vi "Get_Ch_data_from_file.vi"(0 "Filename":path, 9 "Channel names":string[](array[string]), 11 "Start of read offset (chars.: 0)":i32, 12 "Averaging Time(s)":dbl=5.0) -> (4 "exists?":bool, 6 "File Channels":string[](array[string]), 10 "Times":dbl[](array[numeric]) format="%.2f", 15 "Ch Data":dbl[][](array[numeric]) format="%.2f")   [LabVIEW 2015]
uses:
  <vilib>/Analysis/baseanly.llb/Mean (DBL).vi
  <vilib>/Analysis/NI_AALBase.lvlib
panel:
  in  "stop":bool
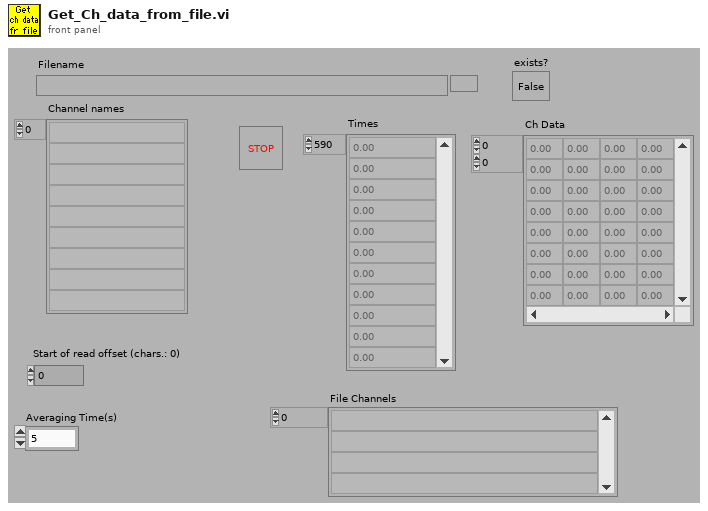
[diagram p1: front panel]
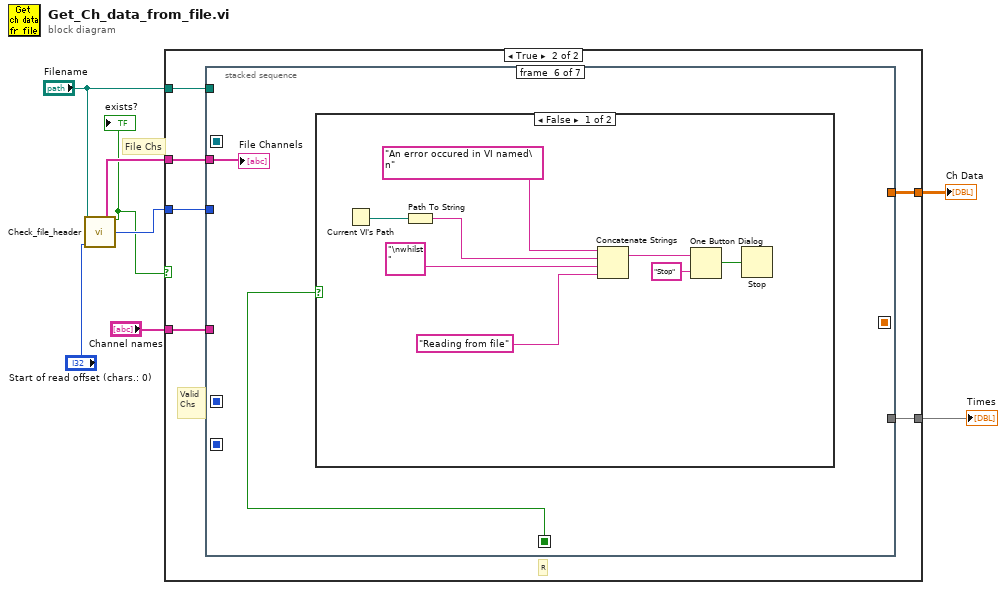
[diagram p0: block diagram]
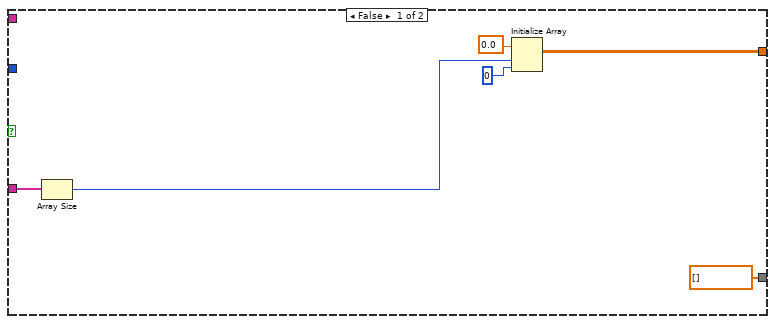
[diagram p2: hidden frame]
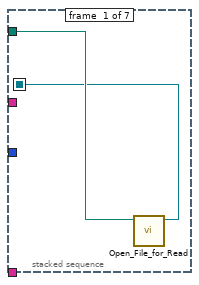
[diagram p3: hidden frame]
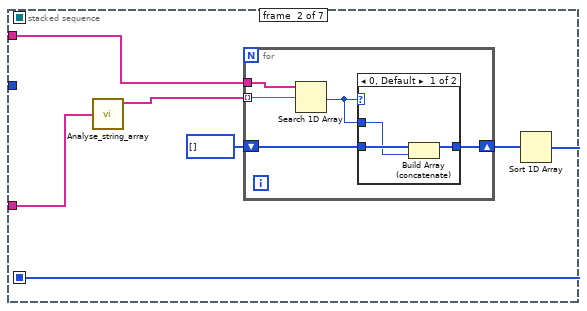
[diagram p4: hidden frame]
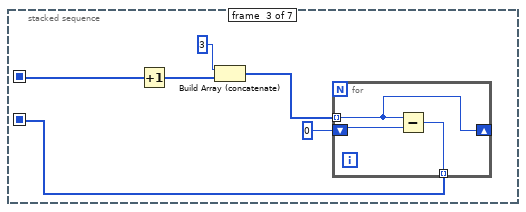
[diagram p6: hidden frame]
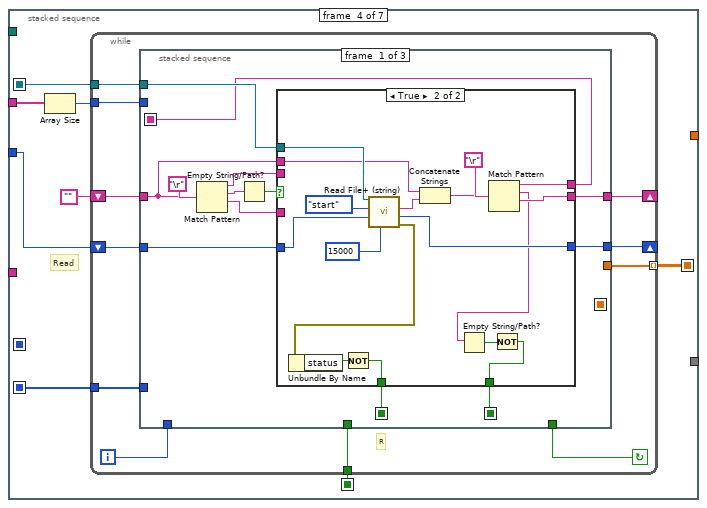
[diagram p7: hidden frame]
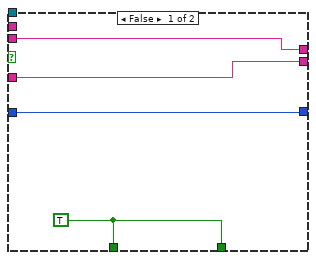
[diagram p8: hidden frame]
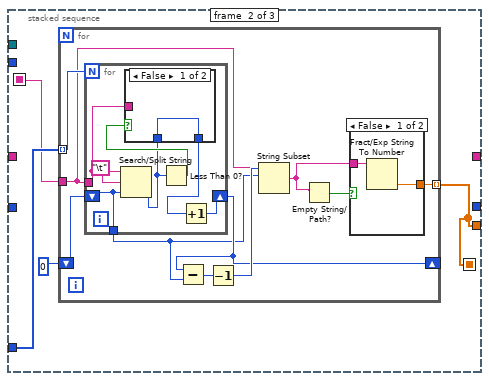
[diagram p9: hidden frame]
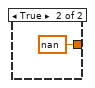
[diagram p10: hidden frame]
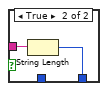
[diagram p11: hidden frame]
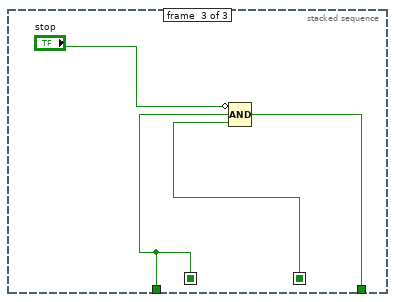
[diagram p12: hidden frame]
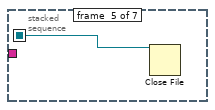
[diagram p13: hidden frame]
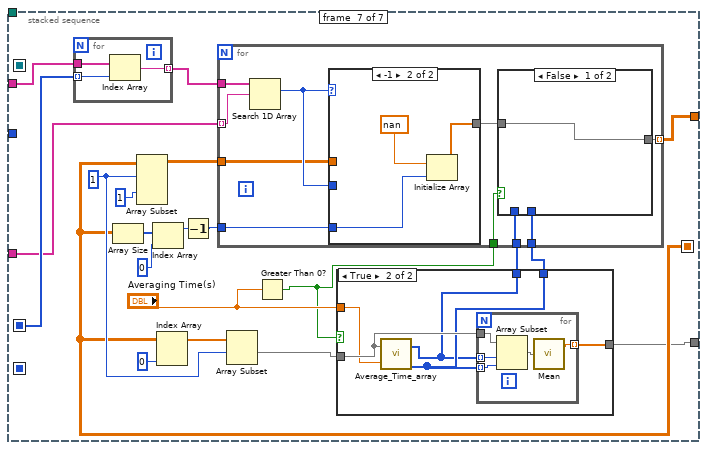
[diagram p15: hidden frame]
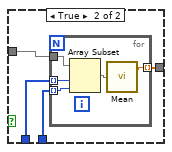
[diagram p17: hidden frame]
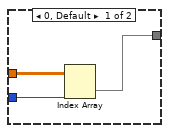
[diagram p18: hidden frame]
diagram:
  # "File Chs"
  n1 = call "Check_file_header.vi"("Filename"="Filename", "Start of read offset (chars.: 0)"="Start of read offset (chars.: 0)") -> ("File Channels"=w7:string[], "exists?"=w4:bool, "Start of data (bytes)"=w8:i32)  [unwired: 2 in, 9 out]
  "exists?" <- w4
  n2 = case shown="True" w4 {
    tunnel: w8 -> [_ w19]
    tunnel: w7 -> [_ w18]
    tunnel: "Filename" -> [_ w20]
    tunnel: [w9 w16] -> w3
    tunnel: [dbl[] [] w15] -> w2
    tunnel: "Channel names" -> [w11 w17]
    frame False {
      n3 = Array Size(array=w11) -> (size(s)=w10:i32)
      n4 = Initialize Array(0.0, w10, 0 ("Dimension Size")) -> (w9:dbl[][])
    }
    frame True {
      # "Valid\nChs"
      # "R"
      n5 = stacked-sequence {
        seq-local: [w21 _ _ _ _ _ _] -> [_ _ _ w53 w131 _ _]
        seq-local: [_ _ _ w50 _ _ _] -> [_ _ _ _ _ w133 _]
        seq-local: [_ _ _ w48 _ _ _] -> [_ _ _ _ _ _ w153]
        seq-local: [_ _ w41 _ _ _ _] -> [_ _ _ w47 _ _ _]
        seq-local: [_ w25 _ _ _ _ _] -> [_ _ w39 _ _ _ w158]
        tunnel: w20 -> [w22 _ _ _ _ _ _]
        tunnel: w19 -> [_ _ _ w52 _ _ _]
        tunnel: w18 -> [_ w28 _ w49 _ w132 w157]
        tunnel: w17 -> [_ w24 _ _ _ _ w156]
        tunnel: [_ _ _ _ _ _ w149] -> w16
        tunnel: [_ _ _ _ _ _ w147] -> w15
        frame #0 {
          n6 = call "Open_File_for_Read.vi"("file path"=w22) -> ("refnum"=w21:refnum<file>)  [unwired: 1 in, 9 out]
        }
        frame #1 {
          n7 = call "Analyse_string_array.vi"("String array"=w24) -> ("Unique strings"=w23:string[])  [unwired: 2 out]
          n8 = for {
            tunnel: w28 -> [w33]
            tunnel: w23 -> [w32] mode=indexing
            shift-right: [w30] -> w26
            shift-left: i32[] [] -> [w31]
            n9 = Search 1D Array(1D array=w33, element=w32) -> (index of element=w29:i32)  [unwired: 1 out]
            n10 = case shown="0, Default" w29 {
              tunnel: w31 -> [w36 w37]
              tunnel: [w34 w37] -> w30
              tunnel: w29 -> [w35 _]
              frame 0, Default {
                n11 = Build Array (concatenate)(w36, w35) -> (w34:i32[])
              }
              frame -1 {
              }
            }
          }
          n12 = Sort 1D Array(array=w26) -> (sorted array=w25:i32[])
        }
        frame #2 {
          n13 = Increment(x=w39) -> (x+1=w38:i32[])
          n14 = Build Array (concatenate)(3 ("t"), w38) -> (w40:i32[])
          n15 = for {
            shift-right: [w45] -> _
            shift-left: 0 -> [w46]
            tunnel: w40 -> [w45] mode=indexing
            tunnel: [w44] -> w41 mode=indexing
            n16 = Subtract(x=w45, y=w46) -> (x-y=w44:i32)
          }
        }
        frame #3 {
          # "Read"
          n17 = Array Size(array=w49) -> (size(s)=w51:i32)
          n18 = while {
            tunnel: w47 -> [w56]
            tunnel: [w58] -> w48 mode=indexing
            tunnel: [w59] -> w50
            tunnel: w51 -> [w60]
            tunnel: w53 -> [w62]
            shift-left: w52 -> [w64]
            shift-right: [w63] -> _
            shift-left: "" -> [w65]
            shift-right: [w61] -> _
            i -> [w57]
            stop <- w55 continue-if-true
            # "R"
            n19 = stacked-sequence {
              seq-local: [w67 _ _] -> [_ w101 _]
              seq-local: [w68 _ _] -> [_ _ w127]
              seq-local: [w69 _ _] -> [_ _ w128]
              seq-local: [_ w100 _] -> [_ _ _]
              tunnel: w65 -> [w72 _ _]
              tunnel: w64 -> [w75 _ _]
              tunnel: [w74 _ _] -> w63
              tunnel: w62 -> [w73 _ _]
              tunnel: [w71 _ _] -> w61
              tunnel: w60 -> [_ _ _]
              tunnel: [_ _ w129] -> w55
              tunnel: [_ _ w128] -> w59
              tunnel: [_ w100 _] -> w58
              tunnel: w57 -> [_ _ _]
              tunnel: w56 -> [_ w103 _]
              frame #0 {
                n20 = Match Pattern(string=w72, regular expression="\r") -> (before substring=w66:string, match substring=w77:string, after substring=w70:string)  [unwired: 2 out]
                n21 = Empty String/Path?(string/path=w77) -> (empty?=w76:bool)
                n22 = case shown="True" w76 {
                  tunnel: w75 -> [w82 w98]
                  tunnel: [w82 w96] -> w74
                  tunnel: w73 -> [_ w95]
                  tunnel: w72 -> [_ w93]
                  tunnel: [w81 w90] -> w71
                  tunnel: w70 -> [w81 _]
                  tunnel: [w80 w86] -> w69
                  tunnel: [w80 w84] -> w68
                  tunnel: [w79 w83] -> w67
                  tunnel: w66 -> [w79 _]
                  frame False {
                    w80 = TRUE
                  }
                  frame True {
                    n23 = call <vilib>:"Read File+ (string).vi"("count"=15000, "pos offset (bytes:0)"=w98, "pos mode (rel. to current:2)"=enum16{"start", "end", "current"}."start", "refnum"=w95) -> ("error out"=w88:errorcluster, "mark after read (bytes)"=w96:i32, "string"=w94:string)  [unwired: 1 in, 4 out]
                    n24 = Unbundle By Name(w88) -> ("status"=w87:bool)
                    n25 = Not(x=w87) -> (.not. x?=w86:bool)
                    n26 = Concatenate Strings(w93, w94) -> (w91:string)
                    n27 = Match Pattern(string=w91, regular expression="\r") -> (before substring=w83:string, match substring=w89:string, after substring=w90:string)  [unwired: 2 out]
                    n28 = Empty String/Path?(string/path=w89) -> (empty?=w85:bool)
                    n29 = Not(x=w85) -> (.not. x?=w84:bool)
                  }
                }
              }
              frame #1 {
                n30 = for {
                  tunnel: w103 -> [w113] mode=indexing
                  tunnel: [w111] -> w100 mode=indexing
                  shift-right: [w105] -> _
                  shift-left: 0 -> [w110]
                  tunnel: w101 -> [w106]
                  n31 = for {
                    N: w113 -> [_]
                    shift-right: [w121] -> w105
                    shift-left: w110 -> [w122]
                    tunnel: w106 -> [w119]
                    tunnel: [w122] -> w104
                    n32 = Search/Split String(string=w119, search string/char (-)="\t", offset (0)=w122) -> (offset of match=w117:i32)  [unwired: 2 out]
                    n33 = Less Than 0?(x=w117) -> (x < 0?=w120:bool)
                    n34 = case shown="False" w120 {
                      tunnel: w119 -> [_ w126]
                      tunnel: [w124 w125] -> w118
                      tunnel: w117 -> [w124 _]
                      frame False {
                      }
                      frame True {
                        n35 = String Length(string=w126) -> (length=w125:i32)
                      }
                    }
                    n36 = Increment(x=w118) -> (x+1=w121:i32)
                  }
                  n37 = Subtract(x=w105, y=w104) -> (x-y=w109:i32)
                  n38 = Decrement(x=w109) -> (x-1=w108:i32)
                  n39 = String Subset(string=w106, offset (0)=w104, length (rest)=w108) -> (substring=w107:string)
                  n40 = Empty String/Path?(string/path=w107) -> (empty?=w112:bool)
                  n41 = case shown="False" w112 {
                    tunnel: w107 -> [w115 _]
                    tunnel: [w114 nan] -> w111
                    frame False {
                      n42 = Fract/Exp String To Number(string=w115) -> (number=w114:dbl)  [unwired: 4 out]
                    }
                    frame True {
                    }
                  }
                }
              }
              frame #2 {
                n43 = Compound Arithmetic op=AND(invert "stop", w128, w127) -> (w129:bool)
              }
            }
          }
        }
        frame #4 {
          n44 = Close File(refnum=w131) -> ()  [unwired: 1 in, 2 out]
        }
        frame #5 {
          n45 = case shown="False" w133 {
            frame False {
              n46 = Current VI's Path() -> (path=w134:path)
              n47 = Path To String(path=w134) -> (string=w140:string)
              n48 = Concatenate Strings("An error occured in VI named\n", w140, "\nwhilst ", "Reading from file") -> (w138:string)
              n49 = One Button Dialog(message=w138, button name ("OK")="Stop") -> (true=w136:bool)
              n50 = Stop(stop? (T)=w136) -> ()
            }
            frame True {
            }
          }
          "File Channels" <- w132
        }
        frame #6 {
          w159 = 1
          n51 = for {
            tunnel: w158 -> [w176] mode=indexing
            tunnel: w157 -> [w175]
            tunnel: [w174] -> w155 mode=indexing
            n52 = Index Array(array=w175, index=w176) -> (element=w174:string)
          }
          n53 = Array Size(array=w153) -> (size(s)=w152:i32[])
          n54 = Array Subset(array=w153, index (row)=w159, index (col)=1) -> (w154:dbl[][])  [unwired: 2 in]
          n55 = Index Array(array=w152, index=0 ("Index")) -> (element=w150:i32)
          n56 = Index Array(array=w153, index (col)=0) -> (element=w160:dbl[])  [unwired: 1 in]
          n57 = Decrement(x=w150) -> (x-1=w148:i32)
          n58 = Array Subset(array=w160, index=w159) -> (w142:dbl[])  [unwired: 1 in]
          n59 = Greater Than 0?(x="Averaging Time(s)") -> (x > 0?=w143:bool)
          n60 = case shown="True" w143 {
            tunnel: w142 -> [w163 w168]
            tunnel: [w163 w167] -> w147
            tunnel: [_ w164] -> w146
            tunnel: [_ w166] -> w145
            tunnel: "Averaging Time(s)" -> [_ w165]
            frame False {
            }
            frame True {
              n61 = call "Average_Time_array.vi"("Average TIme (seconds)"=w165, "Centre Time in Seconds"=w168) -> ("Length"=w166:i32[], "Start"=w164:i32[])
              n62 = for {
                tunnel: w168 -> [w173]
                tunnel: w164 -> [w172] mode=indexing
                tunnel: w166 -> [w171] mode=indexing
                tunnel: [w169] -> w167 mode=indexing
                n63 = Array Subset(array=w173, index=w172, length=w171) -> (w170:dbl[])
                n64 = call-poly <vilib>:"Mean.vi"("X"=w170) -> ("mean"=w169:dbl)  [unwired: 1 out]
              }
            }
          }
          n65 = for {
            tunnel: w156 -> [w186] mode=indexing
            tunnel: w155 -> [w185]
            tunnel: w154 -> [w183]
            tunnel: [w178] -> w149 mode=indexing
            tunnel: w148 -> [w182]
            tunnel: w146 -> [w180]
            tunnel: w145 -> [w179]
            tunnel: w143 -> [w177]
            n66 = Search 1D Array(1D array=w185, element=w186) -> (index of element=w184:i32)  [unwired: 1 out]
            n67 = case shown="-1" w184 {
              tunnel: w184 -> [w197 _]
              tunnel: w183 -> [w199 _]
              tunnel: [w198 w201] -> w181
              tunnel: w182 -> [_ w200]
              frame 0, Default {
                n68 = Index Array(array=w199, index (col)=w197) -> (element=w198:dbl[])  [unwired: 1 in]
              }
              frame -1 {
                n69 = Initialize Array(nan ("Number"), w200) -> (w201:dbl[])
              }
            }
            n70 = case shown="False" w177 {
              tunnel: w181 -> [w187 w191]
              tunnel: w180 -> [_ w190]
              tunnel: w179 -> [_ w189]
              tunnel: [w187 w188] -> w178
              frame False {
              }
              frame True {
                n71 = for {
                  tunnel: w191 -> [w196]
                  tunnel: w190 -> [w195] mode=indexing
                  tunnel: w189 -> [w194] mode=indexing
                  tunnel: [w192] -> w188 mode=indexing
                  n72 = Array Subset(array=w196, index=w195, length=w194) -> (w193:dbl[])
                  n73 = call-poly <vilib>:"Mean.vi"("X"=w193) -> ("mean"=w192:dbl)  [unwired: 1 out]
                }
              }
            }
          }
        }
      }
    }
  }
  "Ch Data" <- w3
  "Times" <- w2
